vi "Func-엑셀 데이터를 그래프로 출력.vi"() -> ()   [LabVIEW 2015] (continued)
  in  "X축-1열":string="시간(m)\n1.23\n1.4\n1.56\n1.73\n1.9\n2.06\n2.23\n2.4\n2.56\n2.73\n2.9\n3.07\n3.23\n3.4\n3.56\n3.73\n3.91\n4.07\n4.24\n4.41\n4.57\n4.74\n4.91\n5.07\n5.24\n5.41\n5.57\n5.74\n5.91\n6.07\n6.24\n6.41\n6.57\n6.74\n6.91\n7.07\n7.24\n7.41\n7.57\n7.74\n7.91\n8.07\n8.24\n8.41\n8.41\n8.43\n8.44\n8.46\n8.48\n8.49\n8.51\n8.53\n8.54\n8.56\n8.58\n8.59\n8.61\n8.63\n8.65\n8.66\n8.68\n8.69\n8.71\n8.73\n8.74\n8.76\n8.78\n8.79\n8.81\n8.83\n8.84\n8.86\n8.88\n8.89\n8.91\n8.93\n8.94\n8.96\n8.98\n9\n9.01\n9.03\n9.04\n9.06\n9.08\n9.1\n9.11\n9.13\n9.14\n9.16\n9.18\n9.19\n9.21\n9.23\n9.25\n9.26\n9.28\n9.29\n9.31\n9.33\n9.35\n9.36\n9.38\n9.39\n9.41\n9.43\n9.44\n9.46\n9.48\n9.49\n9.51\n9.53\n9.54\n9.56\n9.58\n9.59\n9.61\n9.63\n9.64\n9.66\n9.68\n9.7\n9.71\n9.73\n9.74\n9.76\n9.78\n9.79\n9.81\n9.83\n9.84\n9.86\n9.88\n9.9\n9.91\n9.93\n9.94\n9.96\n9.98\n9.99\n10.01\n10.03\n10.04\n10.06\n10.08\n10.09\n10.11\n10.13\n10.14\n10.16\n10.18\n10.19\n10.21\n10.23\n10.24\n10.26\n10.28\n10.29\n10.31\n10.33\n10.34\n10.36\n10.38\n10.39\n10.41\n10.43\n10.44\n10.46\n10.48\n10.49\n10.51\n10.53\n10.54\n10.56\n10.58\n10.59\n10.61\n10.63\n10.64\n10.66\n10.68\n10.69\n10.71\n10.73\n10.74\n10.76\n10.78\n10.79\n10.81\n10.83\n10.84\n10.86\n10.88\n10.89\n10.91\n10.93\n10.94\n10.96\n10.98\n10.99\n11.01\n11.03\n11.04\n11.06\n11.08\n11.09\n11.11\n11.13\n11.14\n11.16\n11.18\n11.19\n11.21\n11.23\n11.24\n11.26\n11.28\n11.29\n11.31\n11.33\n11.34\n11.36\n11.38\n11.39\n11.41\n11.43\n11.44\n11.46\n11.48\n11.49\n11.51\n11.53\n11.54\n11.56\n11.58\n11.59\n11.61\n11.63\n11.64\n11.66\n11.68\n11.69\n11.71\n11.73\n11.74\n11.76\n11.78\n11.79\n11.81\n11.83\n11.85\n11.86\n11.88\n11.89\n11.91\n11.93\n11.94\n11.96\n11.98\n11.99\n12.01\n12.03\n12.04\n12.06\n12.08\n12.1\n12.11\n12.13\n12.14\n12.16\n12.18\n12.2\n12.21\n12.23\n12.24\n12.26\n12.28\n12.29\n12.31\n12.33\n12.35\n12.36\n12.38\n12.39\n12.41\n12.43\n12.45\n12.46\n12.48\n12.49\n12.51\n12.53\n12.55\n12.56\n12.58\n12.59\n12.61\n12.63\n12.64\n12.66\n12.68\n12.7\n12.71\n12.73\n12.74\n12.76\n12.78\n12.79\n12.81\n12.83\n12.84\n12.86\n12.88\n12.89\n12.91\n12.93\n12.94\n12.96\n12.98\n12.99\n13.01\n13.03\n13.04\n13.06\n13.08\n13.09\n13.11\n13.13\n13.14\n13.16\n13.18\n13.19\n13.21\n13.23\n13.24\n13.26\n13.28\n13.29\n13.31\n13.33\n13.34\n13.36\n13.38\n13.39\n13.41\n13.43\n13.44\n13.46\n13.48\n13.49\n13.51\n13.53\n13.54\n13.56\n13.58\n13.59\n13.61\n13.63\n13.64\n13.66\n13.68\n13.69\n13.71\n13.73\n13.74\n13.76\n13.78\n13.79\n13.81\n13.83\n13.84\n13.86\n13.88\n13.89\n13.91\n13.93\n13.94\n13.96\n13.98\n13.99\n14.01\n14.03\n14.04\n14.06\n14.08\n14.09\n14.11\n14.13\n14.14\n14.16\n14.18\n14.19\n14.21\n14.23\n14.24\n14.26\n14.28\n14.29\n14.31\n14.33\n14.34\n14.36\n14.38\n14.39\n14.41\n14.43\n14.44\n14.46\n14.48\n14.49\n14.51\n14.53\n14.54\n14.56\n14.58\n14.6\n14.61\n14.63\n14.64\n14.66\n14.68\n14.69\n14.71\n14.73\n14.74\n14.76\n14.78\n14.79\n14.81\n14.83\n14.84\n14.86\n14.88\n14.89\n14.91\n14.93\n14.95\n14.96\n14.98\n14.99\n15.01\n15.03\n15.04\n15.06\n15.08\n15.09\n15.11\n15.13\n15.14\n15.16\n15.18\n15.2\n15.21\n15.23\n15.24\n15.26\n15.28\n15.3\n15.31\n15.33\n15.34\n15.36\n15.38\n15.39\n15.41\n15.43\n15.44\n15.46\n15.48\n15.49\n15.51\n15.53\n15.54\n15.56\n15.58\n15.59\n15.61\n15.63\n15.65\n15.66\n15.68\n15.69\n15.71\n15.73\n15.74\n15.76\n15.78\n15.79\n15.81\n15.83\n15.84\n15.86\n15.88\n15.89\n15.91\n15.93\n15.94\n15.96\n15.98\n16\n16.01\n16.03\n16.04\n16.06\n16.08\n16.09\n16.11\n16.13\n16.14\n16.16\n16.18\n16.19\n16.21\n16.23\n16.25\n16.26\n16.28\n16.29\n16.31\n16.33\n16.34\n16.36\n16.38\n16.39\n16.41\n16.43\n16.44\n16.46\n16.48\n16.5\n16.51\n16.53\n16.54\n16.56\n16.58\n16.59\n16.61\n16.63\n16.64\n16.66\n16.68\n16.69\n16.71\n16.73\n16.74\n16.76\n16.78\n16.79\n16.81\n16.83\n16.84\n16.86\n16.88\n16.89\n16.91\n16.93\n16.94\n16.96\n16.98\n16.99\n17.01\n17.03\n17.04\n17.06\n17.08\n17.09\n17.11\n17.13\n17.14\n17.16\n17.18\n17.19\n17.21\n17.23\n17.24\n17.26\n17.28\n17.29\n17.31\n17.33\n17.34\n17.36\n17.38\n17.39\n17.41\n17.43\n17.44\n17.46\n17.48\n17.49\n17.51\n17.53\n17.54\n17.56\n17.58\n17.59\n17.61\n17.63\n17.64\n17.66\n17.68\n17.7\n17.71\n17.73\n17.74\n17.76\n17.78\n17.79\n17.81\n17.83\n17.84\n17.86\n17.88\n17.89\n17.91\n17.93\n17.94\n17.96\n17.98\n17.99\n18.01\n18.03\n18.05\n18.06\n18.08\n18.09\n18.11\n18.13\n18.14\n18.16\n18.18\n18.19\n18.21\n18.23\n18.24\n18.26\n18.28\n18.29\n18.31\n18.33\n18.34\n18.36\n18.38\n18.4\n18.41\n18.43\n18.44\n18.46\n18.48\n18.5\n18.51\n18.53\n18.54\n18.56\n18.58\n18.59\n18.61\n18.63\n18.65\n18.66\n18.68\n18.69\n18.71\n18.73\n18.75\n18.76\n18.78\n18.79\n18.81\n18.83\n18.84\n18.86\n18.88\n18.89\n18.91\n18.93\n18.94\n18.96\n18.98\n18.99\n19.01\n19.03\n19.04\n19.06\n19.08\n19.09\n19.11\n19.13\n19.14\n19.16\n19.18\n19.19\n19.21\n19.23\n19.24\n19.26\n19.28\n19.29\n19.31\n19.33\n19.34\n19.36\n19.38\n19.39\n19.41\n19.43\n19.44\n19.46\n19.48\n19.49\n19.51\n19.53\n19.54\n19.56\n19.58\n19.59\n19.61\n19.63\n19.64\n19.66\n19.68\n19.69\n19.71\n19.73\n19.74\n19.76\n19.78\n19.79\n19.81\n19.83\n19.84\n19.86\n19.88\n19.89\n19.91\n19.93\n19.94\n19.96\n19.98\n19.99\n20.01\n20.03\n20.04\n20.06\n20.08\n20.09\n20.11\n20.13\n20.14\n20.16\n20.18\n20.19\n20.21\n20.23\n20.24\n20.26\n20.28\n20.29\n20.31\n20.33\n20.34\n20.36\n20.38\n20.39\n20.41\n20.43\n20.44\n20.46\n20.48\n20.49\n20.51\n20.53\n20.54\n20.56\n20.58\n20.59\n20.61\n20.63\n20.64\n20.66\n20.68\n20.69\n20.71\n20.73\n20.74\n20.76\n20.78\n20.79\n20.81\n20.83\n20.84\n20.86\n20.88\n20.89\n20.91\n20.93\n20.94\n20.96\n20.98\n20.99\n21.01\n21.03\n21.04\n21.06\n21.08\n21.09\n21.11\n21.13\n21.15\n21.16\n21.18\n21.19\n21.21\n21.23\n21.25\n21.26\n21.28\n21.29\n21.31\n21.33\n21.34\n21.36\n21.38\n21.39\n21.41\n21.43\n21.44\n21.46\n21.48\n21.5\n21.51\n21.53\n21.54\n21.56\n21.58\n21.59\n21.61\n21.63\n21.64\n21.66\n21.68\n21.69\n21.71\n21.73\n21.75\n21.76\n21.78\n21.79\n21.81\n21.83\n21.85\n21.86\n21.88\n21.89\n21.91\n21.93\n21.95\n21.96\n21.98\n21.99\n22.01\n22.03\n22.04\n22.06\n22.08\n22.09\n22.11\n22.13\n22.14\n22.16\n22.18\n22.2\n22.21\n22.23\n22.24\n22.26\n22.28\n22.29\n22.31\n22.33\n22.34\n22.36\n22.38\n22.39\n22.41\n22.43\n22.45\n22.46\n22.48\n22.49\n22.51\n22.53\n22.54\n22.56\n22.58\n22.59\n22.61\n22.63\n22.64\n22.66\n22.68\n22.69\n22.71\n22.73\n22.74\n22.76\n22.78\n22.8\n22.81\n22.83\n22.84\n22.86\n22.88\n22.89\n22.91\n22.93\n22.94\n22.96\n22.98\n22.99\n23.01\n23.03\n23.04\n23.06\n23.08\n23.09\n23.11\n23.13\n23.14\n23.16\n23.18\n23.19\n23.21\n23.23\n23.24\n23.26\n23.28\n23.29\n23.31\n23.33\n23.34\n23.36\n23.38\n23.39\n23.41\n23.43\n23.44\n23.46\n23.48\n23.49\n23.51\n23.53\n23.54\n23.56\n23.58\n23.59\n23.61\n23.63\n23.64\n23.66\n23.68\n23.69\n23.71\n23.73\n23.74\n23.76\n23.78\n23.79\n23.81\n23.83\n23.84\n23.86\n23.88\n23.89\n23.91\n23.93\n23.94\n23.96\n23.98\n23.99\n24.01\n24.03\n24.04\n24.06\n24.08\n24.09\n24.11\n24.13\n24.14\n24.16\n24.18\n24.19\n24.21\n24.23\n24.25\n24.26\n24.28\n24.29\n24.31\n24.33\n24.34\n24.36\n24.38\n24.39\n24.41\n24.43\n24.44\n24.46\n24.48\n24.49\n24.51\n24.53\n24.54\n24.56\n24.58\n24.6\n24.61\n24.63\n24.64\n24.66\n24.68\n24.7\n24.71\n24.73\n24.74\n24.76\n24.78\n24.79\n24.81\n24.83\n24.85\n24.86\n24.88\n24.89\n24.91\n24.93\n24.95\n24.96\n24.98\n24.99\n25.01\n25.03\n25.05\n25.06\n25.08\n25.09\n25.11\n25.13\n25.14\n25.16\n25.18\n25.2\n25.21\n25.23\n25.24\n25.26\n25.28\n25.29\n25.31\n25.33\n25.34\n25.36\n25.38\n25.39\n25.41\n25.43\n25.44\n25.46\n25.48\n25.5\n25.51\n25.53\n25.54\n25.56\n25.58\n25.59\n25.61\n25.63\n25.64\n25.66\n25.68\n25.69\n25.71\n25.73\n25.74\n25.76\n25.78\n25.79\n25.81\n25.83\n25.84\n25.86\n25.88\n25.89\n25.91\n25.93\n25.94\n25.96\n25.98\n25.99\n26.01\n26.03\n26.04\n26.06\n26.08\n26.09\n26.11\n26.13\n26.14\n26.16\n26.18\n26.19\n26.21\n26.23\n26.24\n26.26\n26.28\n26.29\n26.31\n26.33\n26.34\n26.36\n26.38\n26.39\n26.41\n26.43\n26.44\n26.46\n26.48\n26.49\n26.51\n26.53\n26.54\n26.56\n26.58\n26.59\n26.61\n26.63\n26.64\n26.66\n26.68\n26.69\n26.71\n26.73\n26.74\n26.76\n26.78\n26.79\n26.81\n26.83\n26.84\n26.86\n26.88\n26.89\n26.91\n26.93\n26.94\n26.96\n26.98\n26.99\n27.01\n27.03\n27.04\n27.06\n27.08\n27.09\n27.11\n27.13\n27.14\n27.16\n27.18\n27.19\n27.21\n27.23\n27.24\n27.26\n27.28\n27.29\n27.31\n27.33\n27.34\n27.36\n27.38\n27.39\n27.41\n27.43\n27.45\n27.46\n27.48\n27.49\n27.51\n27.53\n27.54\n27.56\n27.58\n27.59\n27.61\n27.63\n27.64\n27.66\n27.68\n27.7\n27.71\n27.73\n27.74\n27.76\n27.78\n27.8\n27.81\n27.83\n27.84\n27.86\n27.88\n27.89\n27.91\n27.93\n27.94\n27.96\n27.98\n27.99\n28.01\n28.03\n28.05\n28.06\n28.08\n28.09\n28.11\n28.13\n28.15\n28.16\n28.18\n28.19\n28.21\n28.23\n28.24\n28.26\n28.28\n28.29\n28.31\n28.33\n28.34\n28.36\n28.38\n28.39\n28.41\n28.43\n28.44\n28.46\n28.48\n28.49\n28.51\n28.53\n28.54\n28.56\n28.58\n28.59\n28.61\n28.63\n28.64\n28.66\n28.68\n28.69\n28.71\n28.73\n28.74\n28.76\n28.78\n28.79\n28.81\n28.83\n28.84\n28.86\n28.88\n28.89\n28.91\n28.93\n28.94\n28.96\n28.98\n28.99\n29.01\n29.03\n29.04\n29.06\n29.08\n29.09\n29.11\n29.13\n29.14\n29.16\n29.18\n29.19\n29.21\n29.23\n29.24\n29.26\n29.28\n29.29\n29.31\n29.33\n29.34\n29.36\n29.38\n29.39\n29.41\n29.43\n29.44\n29.46\n29.48\n29.49\n29.51\n29.53\n29.54\n29.56\n29.58\n29.59\n29.61\n29.63\n29.64\n29.66\n29.68\n29.69\n29.71\n29.73\n29.74\n29.76\n29.78\n29.79\n29.81\n29.83\n29.84\n29.86\n29.88\n29.89\n29.91\n29.93\n29.94\n29.96\n29.98\n29.99\n30.01\n30.03\n30.04\n30.06\n30.08\n30.09\n30.11\n30.13\n30.14\n30.16\n30.18\n30.2\n30.21\n30.23\n30.24\n30.26\n30.28\n30.29\n30.31\n30.33\n30.34\n30.36\n30.38\n30.39\n30.41\n30.43\n30.44\n30.46\n30.48\n30.49\n30.51\n30.53\n30.55\n30.56\n30.58\n30.59\n30.61\n30.63\n30.64\n30.66\n30.68\n30.69\n30.71\n30.73\n30.74\n30.76\n30.78\n30.79\n30.81\n30.83\n30.84\n30.86\n30.88\n30.9\n30.91\n30.93\n30.94\n30.96\n30.98\n30.99\n31.01\n31.03\n31.04\n31.06\n31.08\n31.09\n31.11\n31.13\n31.15\n31.16\n31.18\n31.19\n31.21\n31.23\n31.25\n31.26\n31.28\n31.29\n31.31\n31.33\n31.34\n31.36\n31.38\n31.39\n31.41\n31.43\n31.44\n31.46\n31.48\n31.49\n31.51\n31.53\n31.54\n31.56\n31.58\n31.59\n31.61\n31.63\n31.64\n31.66\n31.68\n31.7\n31.71\n31.73\n31.74\n31.76\n31.78\n31.79\n31.81\n31.83\n31.85\n31.86\n31.88\n31.89\n31.91\n31.93\n31.94\n31.96\n31.98\n31.99\n32.01\n32.03\n32.04\n32.06\n32.08\n32.09\n32.11\n32.13\n32.14\n32.16\n32.18\n32.19\n32.21\n32.23\n32.24\n32.26\n32.28\n32.29\n32.31\n32.33\n32.34\n32.36\n32.38\n32.39\n32.41\n32.43\n32.44\n32.46\n32.48\n32.49\n32.51\n32.53\n32.54\n32.56\n32.58\n32.59\n32.61\n32.63\n32.64\n32.66\n32.68\n32.69\n32.71\n32.73\n32.74\n32.76\n32.78\n32.79\n32.81\n32.83\n32.84\n32.86\n32.88\n32.89\n32.91\n32.93\n32.94\n32.96\n32.98\n32.99\n33.01\n33.03\n33.04\n33.06\n33.08\n33.09\n33.11\n33.13\n33.14\n33.16\n33.18\n33.19\n33.21\n33.23\n33.24\n33.26\n33.28\n33.29\n33.31\n33.33\n33.34\n33.36\n33.38\n33.39\n33.41\n33.43\n33.44\n33.46\n33.48\n33.49\n33.51\n33.53\n33.54\n33.56\n33.58\n33.59\n33.61\n33.63\n33.65\n33.66\n33.68\n33.69\n33.71\n33.73\n33.74\n33.76\n33.78\n33.79\n33.81\n33.83\n33.84\n33.86\n33.88\n33.89\n33.91\n33.93\n33.94\n33.96\n33.98\n34\n34.01\n34.03\n34.04\n34.06\n34.08\n34.09\n34.11\n34.13\n34.14\n34.16\n34.18\n34.19\n34.21\n34.23\n34.25\n34.26\n34.28\n34.29\n34.31\n34.33\n34.35\n34.36\n34.38\n34.39\n34.41\n34.43\n34.45\n34.46\n34.48\n34.49\n34.51\n34.53\n34.54\n34.56\n34.58\n34.59\n34.61\n34.63\n34.64\n34.66\n34.68\n34.7\n34.71\n34.73\n34.74\n34.76\n34.78\n34.8\n34.81\n34.83\n34.84\n34.86\n34.88\n34.9\n34.91\n34.93\n34.94\n34.96\n34.98\n34.99\n35.01\n35.03\n35.05\n35.06\n35.08\n35.09\n35.11\n35.13\n35.15\n35.16\n35.18\n35.19\n35.21\n35.23\n35.24\n35.26\n35.28\n35.29\n35.31\n35.33\n35.34\n35.36\n35.38\n35.39\n35.41\n35.43\n35.44\n35.46\n35.48\n35.49\n35.51\n35.53\n35.54\n35.56\n35.58\n35.59\n35.61\n35.63\n35.64\n35.66\n35.68\n35.69\n35.71\n35.73\n35.74\n35.76\n35.78\n35.79\n35.81\n35.83\n35.84\n35.86\n35.88\n35.89\n35.91\n35.93\n35.94\n35.96\n35.98\n35.99\n36.01\n36.03\n36.04\n36.06\n36.08\n36.09\n36.11\n36.13\n36.14\n36.16\n36.18\n36.19\n36.21\n36.23\n36.24\n36.26\n36.28\n36.29\n36.31\n36.33\n36.34\n36.36\n36.38\n36.39\n36.41\n36.43\n36.44\n36.46\n36.48\n36.49\n36.51\n36.53\n36.54\n36.56\n36.58\n36.59\n36.61\n36.63\n36.64\n36.66\n36.68\n36.69\n36.71\n36.73\n36.74\n36.76\n36.78\n36.79\n36.81\n36.83\n36.84\n36.86\n36.88\n36.89\n36.91\n36.93\n36.94\n36.96\n36.98\n36.99\n37.01\n37.03\n37.04\n37.06\n37.08\n37.1\n37.11\n37.13\n37.14\n37.16\n37.18\n37.2\n37.21\n37.23\n37.24\n37.26\n37.28\n37.29\n37.31\n37.33\n37.34\n37.36\n37.38\n37.39\n37.41\n37.43\n37.45\n37.46\n37.48\n37.49\n37.51\n37.53\n37.55\n37.56\n37.58\n37.59\n37.61\n37.63\n37.64\n37.66\n37.68\n37.7\n37.71\n37.73\n37.74\n37.76\n37.78\n37.79\n37.81\n37.83\n37.84\n37.86\n37.88\n37.89\n37.91\n37.93\n37.94\n37.96\n37.98\n37.99\n38.01\n38.03\n38.04\n38.06\n38.08\n38.09\n38.11\n38.13\n38.15\n38.16\n38.18\n38.19\n38.21\n38.23\n38.24\n38.26\n38.28\n38.29\n38.31\n38.33\n38.34\n38.36\n38.38\n38.39\n38.41\n38.43\n38.44\n38.46\n38.48\n38.49\n38.51\n38.53\n38.54\n38.56\n38.58\n38.59\n38.61\n38.63\n38.64\n38.66\n38.68\n38.69\n38.71\n38.73\n38.74\n38.76\n38.78\n38.79\n38.81\n38.83\n38.84\n38.86\n38.88\n38.89\n38.91\n38.93\n38.94\n38.96\n38.98\n38.99\n39.01\n39.03\n39.04\n39.06\n39.08\n39.09\n39.11\n39.13\n39.14\n39.16\n39.18\n39.19\n39.21\n39.23\n39.24\n39.26\n39.28\n39.29\n39.31\n39.33\n39.34\n39.36\n39.38\n39.39\n39.41\n39.43\n39.44\n39.46\n39.48\n39.49\n39.51\n39.53\n39.54\n39.56\n39.58\n39.59\n39.61\n39.63\n39.64\n39.66\n39.68\n39.69\n39.71\n39.73\n39.74\n39.76\n39.78\n39.79\n39.81\n39.83\n39.84\n39.86\n39.88\n39.89\n39.91\n39.93\n39.94\n39.96\n39.98\n39.99\n40.01\n40.03\n40.04\n40.06\n40.08\n40.09\n40.11\n40.13\n40.14\n40.16\n40.18\n40.19\n40.21\n40.23\n40.24\n40.26\n40.28\n40.3\n40.31\n40.33\n40.34\n40.36\n40.38\n40.39\n40.41\n40.43\n40.44\n40.46\n40.48\n40.49\n40.51\n40.53\n40.55\n40.56\n40.58\n40.59\n40.61\n40.63\n40.65\n40.66\n40.68\n40.69\n40.71\n40.73\n40.74\n40.76\n40.78\n40.8\n40.81\n40.83\n40.84\n40.86\n40.88\n40.89\n40.91\n40.93\n40.94\n40.96\n40.98\n41\n41.01\n41.03\n41.04\n41.06\n41.08\n41.09\n41.11\n41.13\n41.14\n41.16\n41.18\n41.19\n41.21\n41.23\n41.24\n41.26\n41.28\n41.29\n41.31\n41.33\n41.34\n41.36\n41.38\n41.39\n41.41\n41.43\n41.44\n41.46\n41.48\n41.49\n41.51\n41.53\n41.54\n41.56\n41.58\n41.59\n41.61\n41.63\n41.64\n41.66\n41.68\n41.69\n41.71\n41.73\n41.74\n41.76\n41.78\n41.79\n41.81\n41.83\n41.84\n41.86\n41.88\n41.89\n41.91\n41.93\n41.94\n41.96\n41.98\n41.99\n42.01\n42.03\n42.04\n42.06\n42.08\n42.09\n42.11\n42.13\n42.14\n42.16\n42.18\n42.19\n42.21\n42.23\n42.24\n42.26\n42.28\n42.29\n42.31\n42.33\n42.34\n42.36\n42.38\n42.39\n42.41\n42.43\n42.44\n42.46\n42.48\n42.49\n42.51\n42.53\n42.54\n42.56\n42.58\n42.59\n42.61\n42.63\n42.64\n42.66\n42.68\n42.69\n42.71\n42.73\n42.74\n42.76\n42.78\n42.79\n42.81\n42.83\n42.84\n42.86\n42.88\n42.89\n42.91\n42.93\n42.94\n42.96\n42.98\n42.99\n43.01\n43.03\n43.05\n43.06\n43.08\n43.09\n43.11\n43.13\n43.14\n43.16\n43.18\n43.19\n43.21\n43.23\n43.24\n43.26\n43.28\n43.3\n43.31\n43.33\n43.34\n43.36\n43.38\n43.4\n43.41\n43.43\n43.44\n43.46\n43.48\n43.49\n43.51\n43.53\n43.54\n43.56\n43.58\n43.59\n43.61\n43.63\n43.65\n43.66\n43.68\n43.69\n43.71\n43.73\n43.75\n43.76\n43.78\n43.79\n43.81\n43.83\n43.84\n43.86\n43.88\n43.89\n43.91\n43.93\n43.94\n43.96\n43.98\n44\n44.01\n44.03\n44.04\n44.06\n44.08\n44.1\n44.11\n44.13\n44.14\n44.16\n44.18\n44.19\n44.21\n44.23\n44.25\n44.26\n44.28\n44.29\n44.31\n44.33\n44.34\n44.36\n44.38\n44.39\n44.41\n44.43\n44.44\n44.46\n44.48\n44.49\n44.51\n44.53\n44.55\n44.56\n44.58\n44.59\n44.61\n44.63\n44.64\n44.66\n44.68\n44.7\n44.71\n44.73\n44.74\n44.76\n44.78\n44.8\n44.81\n44.83\n44.84\n44.86\n44.88\n44.89\n44.91\n44.93\n44.94\n44.96\n44.98\n44.99\n45.01\n45.03\n45.04\n45.06\n45.08\n45.09\n45.11\n45.13\n45.14\n45.16\n45.18\n45.19\n45.21\n45.23\n45.24\n45.26\n45.28\n45.29\n45.31\n45.33\n45.34\n45.36\n45.38\n45.39\n45.41\n45.43\n45.44\n45.46\n45.48\n45.49\n45.51\n45.53\n45.54\n45.56\n45.58\n45.59\n45.61\n45.63\n45.64\n45.66\n45.68\n45.69\n45.71\n45.73\n45.74\n45.76\n45.78\n45.79\n45.81\n45.83\n45.84\n45.86\n45.88\n45.89\n45.91\n45.93\n45.94\n45.96\n45.98\n45.99\n46.01\n46.03\n46.04\n46.06\n46.08\n46.09\n46.11\n46.13\n46.15\n46.16\n46.18\n46.19\n46.21\n46.23\n46.24\n46.26\n46.28\n46.29\n46.31\n46.33\n46.34\n46.36\n46.38\n46.39\n46.41\n46.43\n46.44\n46.46\n46.48\n46.5\n46.51\n46.53\n46.54\n46.56\n46.58\n46.59\n46.61\n46.63\n46.64\n46.66\n46.68\n46.69\n46.71\n46.73\n46.75\n46.76\n46.78\n46.79\n46.81\n46.83\n46.85\n46.86\n46.88\n46.89\n46.91\n46.93\n46.95\n46.96\n46.98\n46.99\n47.01\n47.03\n47.04\n47.06\n47.08\n47.09\n47.11\n47.13\n47.14\n47.16\n47.18\n47.2\n47.21\n47.23\n47.24\n47.26\n47.28\n47.3\n47.31\n47.33\n47.34\n47.36\n47.38\n47.39\n47.41\n47.43\n47.44\n47.46\n47.48\n47.49\n47.51\n47.53\n47.54\n47.56\n47.58\n47.59\n47.61\n47.63\n47.64\n47.66\n47.68\n47.69\n47.71\n47.73\n47.74\n47.76\n47.78\n47.8\n47.81\n47.83\n47.84\n47.86\n47.88\n47.89\n47.91\n47.93\n47.94\n47.96\n47.98\n47.99\n48.01\n48.03\n48.04\n48.06\n48.08\n48.09\n48.11\n48.13\n48.14\n48.16\n48.18\n48.19\n48.21\n48.23\n48.24\n48.26\n48.28\n48.29\n48.31\n48.33\n48.34\n48.36\n48.38\n48.39\n48.41\n48.43\n48.44\n48.46\n48.48\n48.49\n48.51\n48.53\n48.54\n48.56\n64.59\n64.76\n64.93\n65.1\n65.26\n65.43\n65.6\n65.77\n65.94\n66.11\n66.27\n66.44\n66.61\n66.77\n66.94\n67.11\n67.27\n67.44\n67.61\n67.77\n67.94\n68.11\n68.27\n68.44\n68.61\n68.77\n68.94\n69.11\n69.27\n69.44\n69.61\n69.77\n69.94\n70.11\n70.27\n70.44\n70.61\n70.77\n70.94\n71.11\n71.27\n71.44\n71.61\n71.77\n71.94\n72.11\n72.27\n72.44\n72.61\n72.77\n72.94\n73.11\n73.27\n73.44\n73.61\n73.77\n73.94\n74.11\n74.27\n74.44\n74.61\n74.77\n74.94\n75.11\n75.27\n75.44\n75.61\n75.78\n75.95\n76.11\n76.28\n76.45\n76.61\n76.78\n76.95\n77.11\n77.28\n77.45\n77.62\n77.78\n77.95\n78.11\n78.28\n78.45\n78.61\n78.78\n78.95\n79.12\n79.28\n79.45\n79.61\n79.78\n79.95\n80.11\n80.28\n80.45\n80.61\n80.78\n80.95\n81.11\n81.28\n81.45\n81.61\n81.78\n81.95\n82.11\n82.28\n82.45\n82.61\n82.78\n82.95\n83.11\n83.28\n83.45\n83.61\n83.78\n83.95\n84.11\n84.28\n84.45\n84.62\n84.78\n84.95\n85.11\n85.28\n85.45\n85.61\n85.78\n85.95\n86.11\n86.28\n86.45\n86.61\n86.78\n86.95\n87.11\n87.28\n87.45\n87.62\n87.78\n87.95\n88.11\n88.28\n88.45\n88.61\n88.78\n88.95\n89.11\n89.28\n89.45\n89.61\n89.78\n89.95\n90.12\n90.28\n90.45\n90.61\n90.78\n90.95\n91.11\n91.28\n91.45\n91.61\n91.78\n91.95\n92.11\n92.28\n92.45\n92.61\n92.78\n92.95\n93.11\n93.28\n93.45\n93.61\n93.78\n93.95\n94.11\n94.28\n94.45\n94.61\n94.78\n94.95\n95.11\n95.28\n95.45\n95.61\n95.78\n95.95\n96.11\n96.28\n96.45\n96.61\n96.78\n96.95\n97.11\n97.28\n97.45\n97.61\n97.78\n97.95\n98.11\n98.28\n98.45\n98.61\n98.78\n98.95\n99.11\n99.28\n99.45\n99.61\n99.78\n99.95\n100.11\n100.28\n100.45\n100.62\n100.78\n100.95\n101.11\n101.28\n101.45\n101.61\n101.78\n101.95\n102.11\n102.28\n102.45\n102.61\n102.78\n102.95\n103.11\n103.28\n103.45\n103.61\n103.78\n103.95\n104.11\n104.28\n104.45\n104.61\n104.78\n104.95\n105.11\n105.28\n105.45\n105.62\n105.78\n105.95\n106.11\n106.28\n106.45\n106.61\n106.78\n106.95\n107.11\n107.28\n107.45\n107.61\n107.76\n107.78\n107.79\n107.81\n107.83\n107.84\n107.86\n107.88\n107.89\n107.91\n107.93\n107.94\n107.96\n107.98\n108\n108.01\n108.03\n108.04\n108.06\n108.08\n108.09\n108.11\n108.13\n108.14\n108.16\n108.18\n108.19\n108.21\n108.23\n108.24\n108.26\n108.28\n108.29\n108.31\n108.33\n108.35\n108.36\n108.38\n108.39\n108.41\n108.43\n108.44\n108.46\n108.48\n108.49\n108.51\n108.53\n108.54\n108.56\n108.58\n108.59\n108.61\n108.63\n108.64\n108.66\n108.68\n108.7\n108.71\n108.73\n108.74\n108.76\n108.78\n108.8\n108.81\n108.83\n108.84\n108.86\n108.88\n108.89\n108.91\n108.93\n108.94\n108.96\n108.98\n108.99\n109.01\n109.03\n109.05\n109.06\n109.08\n109.09\n109.11\n109.13\n109.15\n109.16\n109.18\n109.2\n109.21\n109.23\n109.24\n109.26\n109.28\n109.29\n109.31\n109.33\n109.34\n109.36\n109.38\n109.4\n109.41\n109.43\n109.44\n109.46\n109.48\n109.5\n109.51\n109.53\n109.54\n109.56\n109.58\n109.59\n109.61\n109.63\n109.64\n109.66\n109.68\n109.69\n109.71\n109.73\n109.75\n109.76\n109.78\n109.79\n109.81\n109.83\n109.84\n109.86\n109.88\n109.89\n109.91\n109.93\n109.94\n109.96\n109.98\n110\n110.01\n110.03\n110.04\n110.06\n110.08\n110.09\n110.11\n110.13\n110.14\n
